vi "CAN_close_all.vi"(8 "Input Error out array":errorcluster[](array[cluster]), 11 "Input CANopen Sessions array":refnum<class "sbCANopenBaseClass.lvclass">[](array[class])) -> ()   [LabVIEW 2024]
uses:
  <vilib>/addons/Maxon Motor/EPOS2 CANopen/CANopen/sbCANopenBaseClass.lvclass
  <vilib>/addons/Maxon Motor/EPOS2 CANopen/EPOS2 Support Files/Typedefs/EPOS2 Control Word PVM.ctl
  <vilib>/addons/Maxon Motor/EPOS2 CANopen/EPOS2 Support Files/Polymorphic SubVIs/Write PDO/EPOS2 Current Mode Write.vi
  <vilib>/addons/Maxon Motor/EPOS2 CANopen/EPOS2 Library.lvlib
panel:
  out "Array of Error out's":errorcluster[](array[cluster])
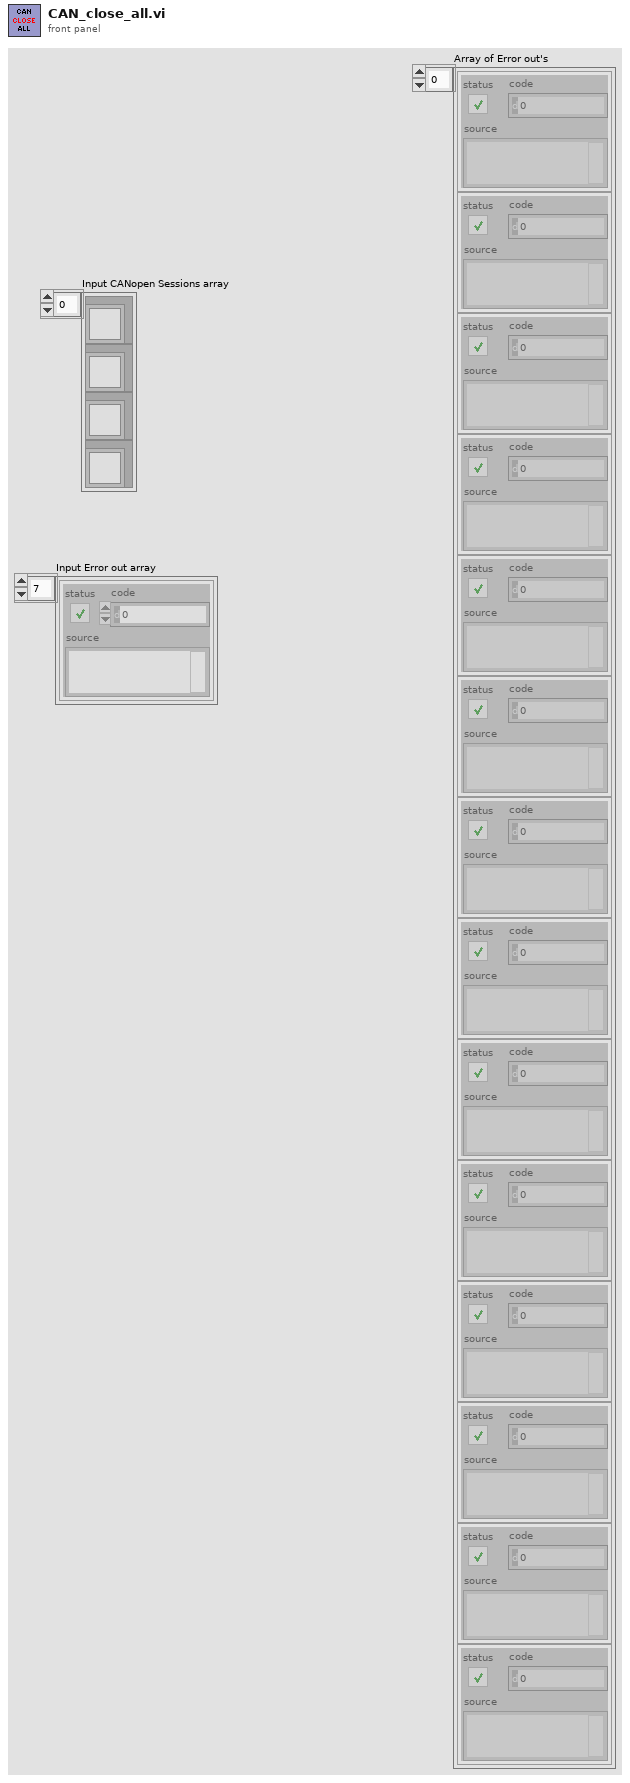
[diagram p1: front panel]
types:
  T1 = typedef "EPOS2 Library.lvlib/EPOS2 Control Word PVM.ctl" = cluster{"Switch On":bool, "Enable Voltage":bool, "Quick Stop":bool, "Enable Operation":bool, "Reserved 0":bool, "Reserved 1":bool, "Reserved 2":bool, "Fault Reset":bool, "Halt":bool}
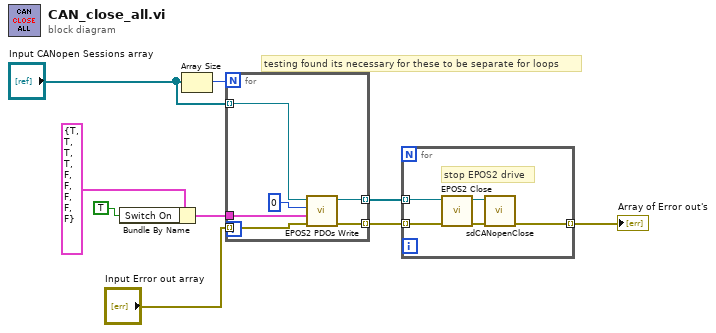
[diagram p0: block diagram]
diagram:
  # "testing found its necessary for these to be separate for loops"
  n1 = Bundle By Name(cluster=T1 {"Switch On"=TRUE, "Enable Voltage"=TRUE, "Quick Stop"=TRUE, "Enable Operation"=TRUE, "Reserved 0"=FALSE, "Reserved 1"=FALSE, "Reserved 2"=FALSE, "Fault Reset"=FALSE, "Halt"=FALSE} ("Control Word"), "Switch On"=TRUE) -> (w4:T1)
  n2 = Array Size(array="Input CANopen Sessions array") -> (size(s)=w9:i32)
  n3 = for {
    N: w9 -> [_]
    tunnel: "Input CANopen Sessions array" -> [w13] mode=indexing
    tunnel: "Input Error out array" -> [w12] mode=indexing
    tunnel: w4 -> [w15]
    tunnel: [w11] -> w3 mode=indexing
    tunnel: [w10] -> w2 mode=indexing
    n4 = call-poly <vilib>:"EPOS2 PDOs Write.vi"("error in"=w12, "Control Word"=w15, "Current"=0, "CANopen Session In"=w13) -> ("error out"=w10:errorcluster, "CANopen Session Out"=w11:refnum<class "sbCANopenBaseClass.lvclass">)  [unwired: 6 in]
  }
  n5 = for {
    tunnel: w3 -> [w18] mode=indexing
    tunnel: w2 -> [w17] mode=indexing
    tunnel: [w16] -> w1 mode=indexing
    # "stop EPOS2 drive"
    n6 = call <vilib>:"EPOS2 Close.vi"("error in"=w17, "CANopen Session In"=w18) -> ("error out"=w19:errorcluster, "CANopen Session Out"=w20:refnum<class "sbCANopenBaseClass.lvclass">)  [unwired: 2 in, 6 out]
    n7 = call-dynamic "sdCANopenClose.vi"("error in (no error)"=w19, "sbCANopenBaseClass in"=w20) -> ("error out"=w16:errorcluster)  [unwired: 8 in, 1 out]
  }
  "Array of Error out's" <- w1
